vi "LAN Reset.vi"(8 "error in":errorcluster, 10 "Node In":string, 11 "VISA resource name":refnum<visa-resource-name>) -> (0 "error out":errorcluster, 2 "Node Out":string, 3 "VISA resource name out":refnum<visa-resource-name>, 4 "Command String":string)   [LabVIEW 2009, in "Keithley 2600 Series.lvlib"]
doc: "This VI resets the LAN interface.\n\n<b>Functions and Attributes Used</b>\nlan.reset()"
uses:
  <instrlib>/Keithley 2600 Series/Keithley 2600 Series.lvlib
panel:
  # "(c) 2008 Keithley Instruments, Inc.  ALL RIGHTS RESERVED."
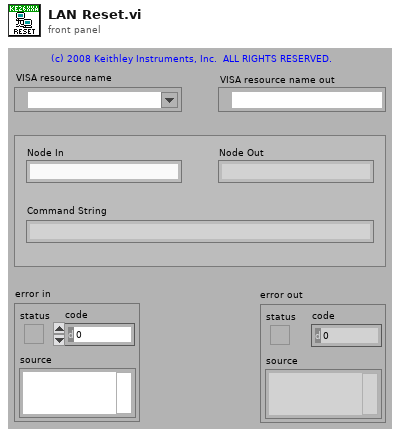
[diagram p1: front panel]
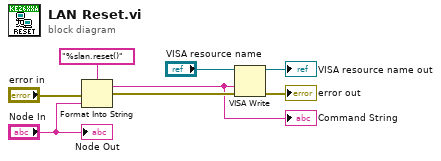
[diagram p0: block diagram]
diagram:
  n1 = Format Into String(format string="%slan.reset()", error in="error in", "Node In") -> (resulting string=w5:string, error out=w8:errorcluster)  [unwired: 1 in]
  "Command String" <- w5
  n2 = VISA Write(VISA resource name="VISA resource name", write buffer=w5, error in (no error)=w8) -> (VISA resource name out=→"VISA resource name out":refnum<visa-resource-name>, error out=→"error out":errorcluster)  [unwired: 1 out]
  "Node Out" <- "Node In"
